vi "Mach1-TestRT-08-16.vi"() -> ()   [LabVIEW 2010]
uses:
  <vilib>/userDefined/High Color/nirio_resource_hc.ctl
  <vilib>/rvi/interface/nirviOpenFPGA/nirviOpenFPGA.xnode
  C:/Users/HAGAR-IV/Desktop/Zeugs/markus/version feb 2012/FPGA Bitfiles/pertrasgcfpga2_FPGATarget_Mach1-Test-08-16_84F9B2AA.lvbitx
  C:/Users/HAGAR-IV/Desktop/HAGAR-V_Steuerung/Users/HAGAR-IV/Desktop/Johnny/pertrasgc fpga/Mach1-Test-08-16.vi
  <vilib>/rvi/ClientSDK/nirviWhatTheDeviceIsDoing.ctl
  <vilib>/rvi/interface/nirviReadWriteControl/nirviReadWriteControl.xnode
  <vilib>/rvi/interface/common/niFpgaNodeNameForErrorReporting.ctl
  <vilib>/rvi/errors/niLvFpgaWhatHappensToTopLevelVI.ctl
  <vilib>/rvi/interface/nirviMethod/nirviMethod.xnode
  <vilib>/rvi/interface/nirviCloseFPGA/nirviCloseFPGA.xnode
  <vilib>/FPGAPlugInAG/cRIO-9114/niLvFpga_Open_cRIO-9114.vi
  <vilib>/rvi/interface/common/dynamic/niFpgaDynamicAddResources.vi
  <vilib>/Utility/error.llb/Error Cluster From Error Code.vi
  <vilib>/rvi/errors/niLvFpgaAdjustHostInterfaceError.vi
  <vilib>/FPGAPlugInAG/Dynamic/niLvFpga_Close_Dynamic.vi
  NiFpgaLv.dll
panel:
  in  "GrapfikLöschen":bool
  out "TempMach2":dbl[](graph)
  out "TempMach1":dbl[](graph)
  in  "2Pos1A":bool
  in  "Fan2":bool
  in  "Fan1":bool
  out "TempMach2":dbl
  out "TempMach1":dbl
  in  "KennlinieMach2":dbl[](array[numeric])=[-254.36, 617.83, -163.64]
  in  "TempMaxMach1":dbl format="%.14g"
  in  "TempMaxMach2":dbl format="%.14g"
  in  "PIDMach2":T1 {"proportional gain (Kc)" format="%.11g"; "integral gain (Kc*Ts/Ti)" format="%.11g"; "derivative gain (Kc*Td/Ts)" format="%.11g"}
  in  "PIDMach1":T1 {"proportional gain (Kc)" format="%.11g"; "integral gain (Kc*Ts/Ti)" format="%.11g"; "derivative gain (Kc*Td/Ts)" format="%.11g"}
  in  "Heizen?Mach2":bool
  in  "Heizen?Mach1":bool
  in  "Abstand zwischen Messungen [us]Mach":u16=20
  in  "wie viele Messwerte?Mach":u16=10
  in  "vor der Messung [us]Mach":u16=3000
  in  "Per[us]Mach":u16=30000
  in  "stop":bool
  in  "KennlinieMach1":dbl[](array[numeric])=[-247.14, 362.24, -56.76]
  in  "TempSPMach1":dbl format="%.14g"
  in  "TempSPMach2":dbl format="%.14g"
  # "Obacht: Hier gehts um\nPRE-MACH 1 und 2!!!"
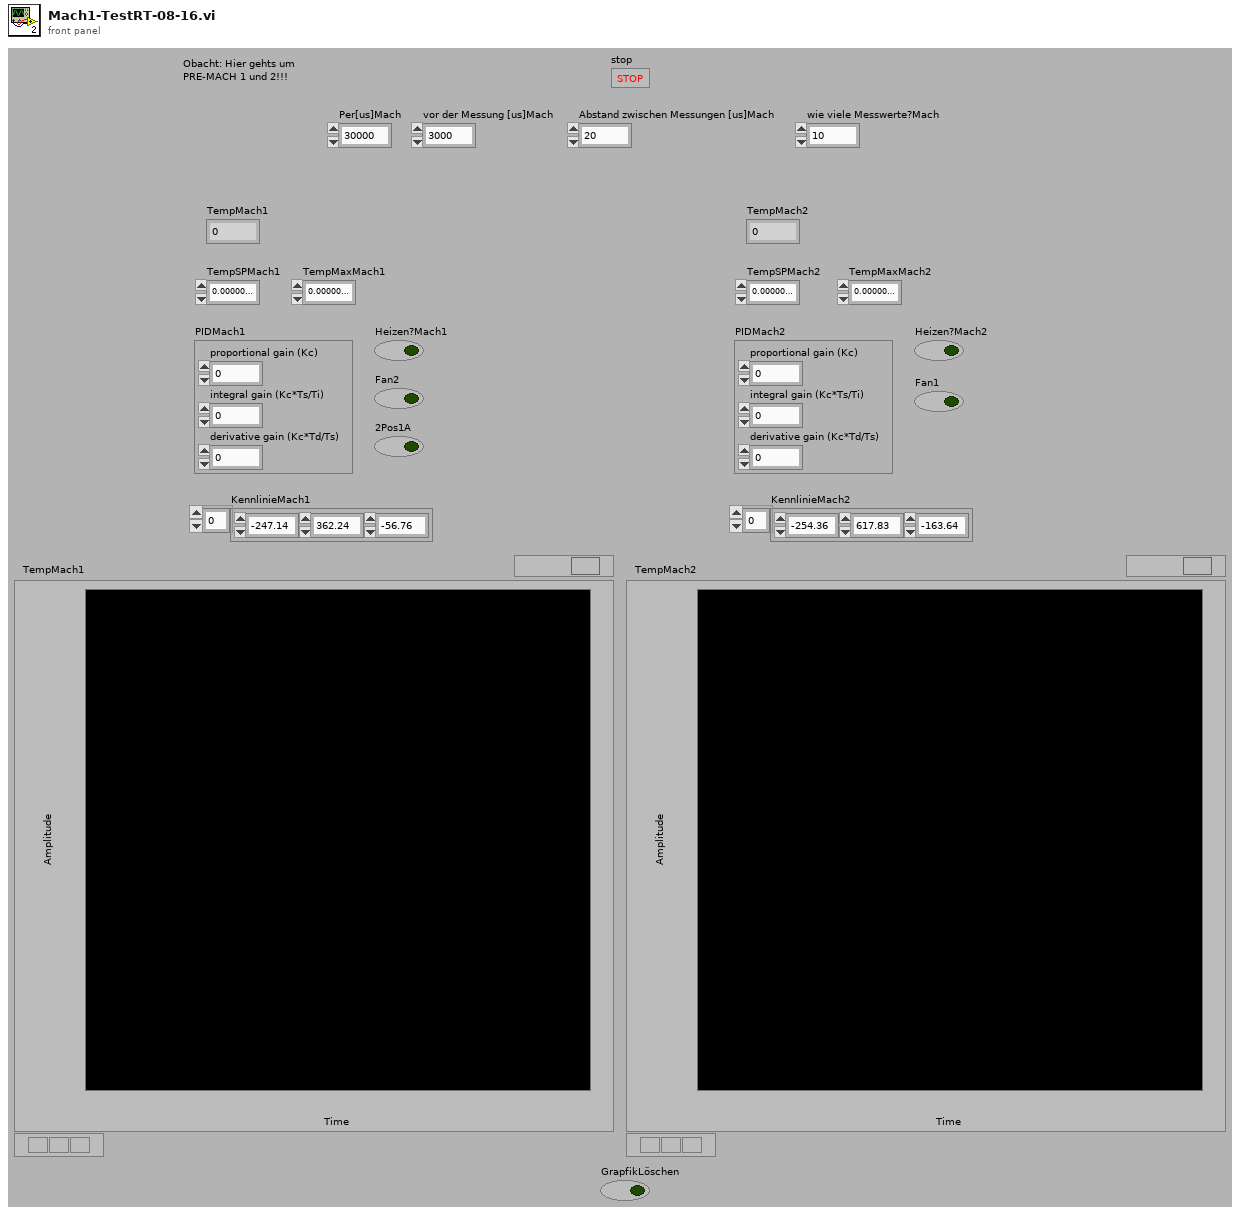
[diagram p1: front panel]
types:
  T1 = cluster{"proportional gain (Kc)":fxp<+/-,16,8>, "integral gain (Kc*Ts/Ti)":fxp<+/-,16,8>, "derivative gain (Kc*Td/Ts)":fxp<+/-,16,8>}
  T2 = typedef "niFpgaNodeNameForErrorReporting.ctl" = enum16{"Open FPGA VI Reference", "Read/Write Control", "Invoke Method: Abort", "Invoke Method: Acknowledge IRQ", "Invoke Method: Download", "Invoke Method: FIFO.Configure", "Invoke Method: FIFO.Read", "Invoke Method: FIFO.Start", "Invoke Method: FIFO.Stop", "Invoke Method: FIFO.Write", "Invoke Method: Reset", "Invoke Method: Run", "Invoke Method: Wait on IRQ", "Close FPGA VI Reference"}
  T3 = typedef "niLvFpgaWhatHappensToTopLevelVI.ctl" = enum16{"top level VI scripted behind XNode", "top level VI inlined behind XNode"}
  T4 = typedef "nirviWhatTheDeviceIsDoing.ctl" = enum32{"nothing", "something other than LabVIEW FPGA", "FPGA interface", "interactive", "emulation"}
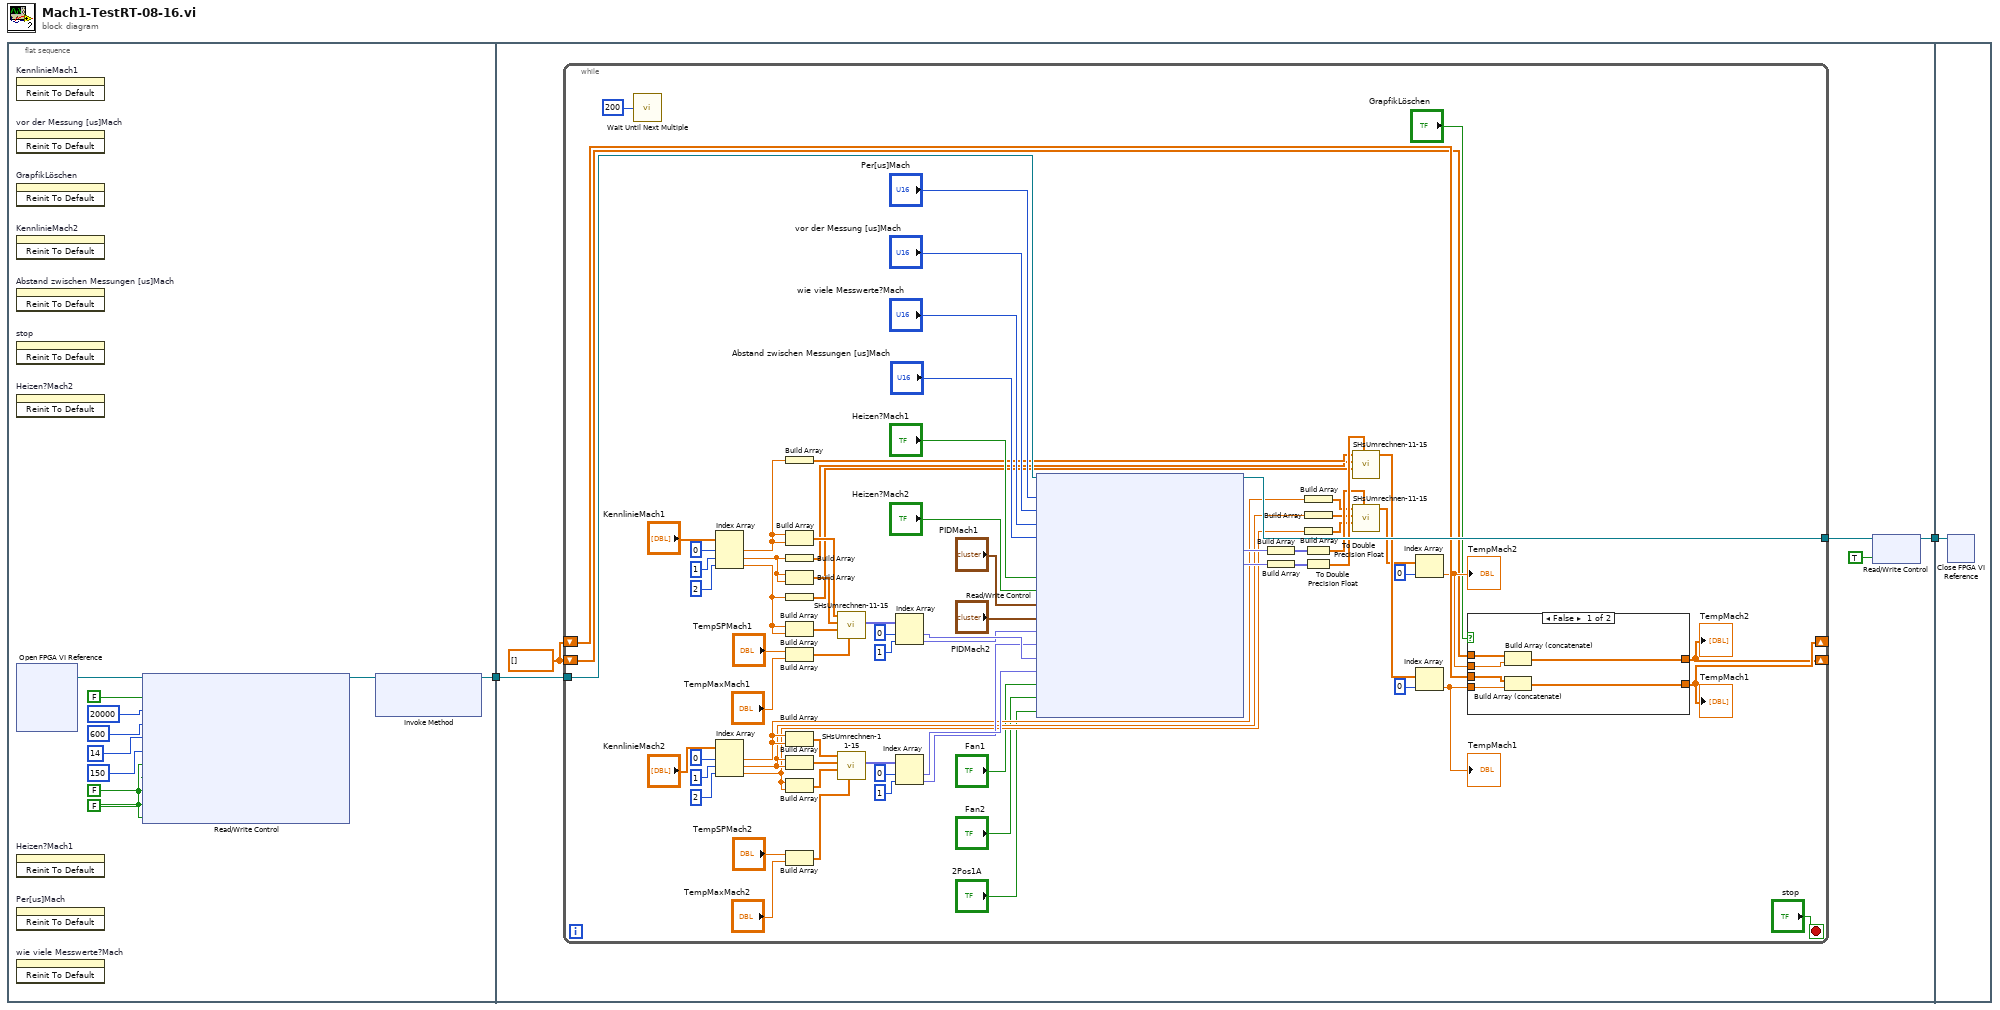
[diagram p0: block diagram]
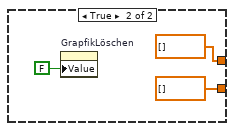
[diagram p2: hidden frame]
diagram:
  n1 = flat-sequence {
    tunnel: [w10] -> w2
    tunnel: w2 -> [w345]
    tunnel: [w342] -> w1
    tunnel: w1 -> [w913]
    frame #0 {
      w3 = FALSE ("Heizen?Mach2")
      n2 = invoke on="KennlinieMach1" class="Arr (strict)" method="Reinit To Default"() -> ()  [unwired: 3 in, 3 out]
      n3 = invoke on="vor der Messung [us]Mach" class="DigNum (strict)" method="Reinit To Default"() -> ()  [unwired: 3 in, 3 out]
      n4 = invoke on="GrapfikLöschen" class="Bool (strict)" method="Reinit To Default"() -> ()  [unwired: 3 in, 3 out]
      n5 = invoke on="KennlinieMach2" class="Arr (strict)" method="Reinit To Default"() -> ()  [unwired: 3 in, 3 out]
      n6 = invoke on="Abstand zwischen Messungen [us]Mach" class="DigNum (strict)" method="Reinit To Default"() -> ()  [unwired: 3 in, 3 out]
      n7 = invoke on="stop" class="Bool (strict)" method="Reinit To Default"() -> ()  [unwired: 3 in, 3 out]
      n8 = invoke on="Heizen?Mach2" class="Bool (strict)" method="Reinit To Default"() -> ()  [unwired: 3 in, 3 out]
      n9 = xnode "Open FPGA VI Reference"() -> ("FPGA VI Reference Out"=w12:refnum<k20>)  [unwired: 2 in, 1 out]
      n10 = invoke on="Heizen?Mach1" class="Bool (strict)" method="Reinit To Default"() -> ()  [unwired: 3 in, 3 out]
      n11 = invoke on="Per[us]Mach" class="DigNum (strict)" method="Reinit To Default"() -> ()  [unwired: 3 in, 3 out]
      n12 = invoke on="wie viele Messwerte?Mach" class="DigNum (strict)" method="Reinit To Default"() -> ()  [unwired: 3 in, 3 out]
      n13 = xnode "Read/Write Control"("FPGA VI Reference In"=w12, "stop"=FALSE, "Per[us]Mach"=u16 20000, "vor der Messung [us]Mach"=u16 600, "wie viele Messwerte?Mach"=u16 14, "Abstand zwischen Messungen [us]Mach"=u16 150, "Heizen?Mach1"=FALSE, "Heizen?Mach2"=w3, "Fan1"=w3, "Fan2"=w3, "2Pos1A"=w3) -> ("FPGA VI Reference Out"=w11:refnum<k20>)  [unwired: 1 in, 1 out]
      n14 = xnode "Invoke Method"("FPGA VI Reference In"=w11) -> ("FPGA VI Reference Out"=w10:refnum<k20>)  [unwired: 2 in, 1 out]
    }
    frame #1 {
      w341 = dbl[] []
      n15 = while {
        tunnel: w345 -> [w458]
        tunnel: [w457] -> w344
        shift-right: [w386] -> _
        shift-left: w341 -> [w390]
        shift-right: [w385] -> _
        shift-left: w341 -> [w388]
        stop <- "stop" stop-if-true
        n16 = call "Wait Until Next Multiple"("Count(mSec)"=u32 200) -> ()  [unwired: 1 out]
        n17 = Index Array(array="KennlinieMach1", index #1=0 ("index"), index #2=1 ("index"), index #3=2 ("index")) -> (element #1=w410:dbl, element #2=w409:dbl, element #3=w408:dbl)
        n18 = Index Array(array="KennlinieMach2", index #1=0 ("index"), index #2=1 ("index"), index #3=2 ("index")) -> (element #1=w402:dbl, element #2=w401:dbl, element #3=w400:dbl)
        n19 = Build Array(w410) -> (w407:dbl[])
        n20 = Build Array(w410, w410) -> (w426:dbl[])
        n21 = Build Array(w409) -> (w406:dbl[])
        n22 = Build Array(w409, w409) -> (w425:dbl[])
        n23 = Build Array(w408) -> (w405:dbl[])
        n24 = Build Array(w408, w408) -> (w424:dbl[])
        n25 = Build Array("TempSPMach1", "TempMaxMach1") -> (w444:dbl[])
        n26 = Build Array(w402, w402) -> (w419:dbl[])
        n27 = Build Array(w401, w401) -> (w418:dbl[])
        n28 = Build Array(w400, w400) -> (w417:dbl[])
        n29 = Build Array("TempSPMach2", "TempMaxMach2") -> (w436:dbl[])
        n30 = call "SHsUmrechnen-11-15.vi"("TemperaturenSH[V]"=w444, "Traps/MachKoeff2"=w424, "Traps/MachKoeff1"=w425, "Traps/MachKoeff0"=w426) -> ("SpannungenSH[V]"=w443:fxp<+/-,16,4>[])  [unwired: 6 in, 1 out]
        n31 = call "SHsUmrechnen-11-15.vi"("TemperaturenSH[V]"=w436, "Traps/MachKoeff2"=w417, "Traps/MachKoeff1"=w418, "Traps/MachKoeff0"=w419) -> ("SpannungenSH[V]"=w433:fxp<+/-,16,4>[])  [unwired: 6 in, 1 out]
        n32 = Index Array(array=w443, index #1=0 ("index"), index #2=1 ("index")) -> (element #1=w440:fxp<+/-,16,4>, element #2=w439:fxp<+/-,16,4>)
        n33 = Index Array(array=w433, index #1=0 ("index"), index #2=1 ("index")) -> (element #1=w432:fxp<+/-,16,4>, element #2=w431:fxp<+/-,16,4>)
        n34 = xnode "Read/Write Control"("FPGA VI Reference In"=w458, "Per[us]Mach"="Per[us]Mach", "vor der Messung [us]Mach"="vor der Messung [us]Mach", "wie viele Messwerte?Mach"="wie viele Messwerte?Mach", "Abstand zwischen Messungen [us]Mach"="Abstand zwischen Messungen [us]Mach", "Heizen?Mach1"="Heizen?Mach1", "Heizen?Mach2"="Heizen?Mach2", "PIDMach1"="PIDMach1", "PIDMach2"="PIDMach2", "Umax[V]Mach1"=w439, "Umax[V]Mach2"=w431, "USetp[V]Mach1"=w440, "USetp[V]Mach2"=w432, "Fan1"="Fan1", "Fan2"="Fan2", "2Pos1A"="2Pos1A") -> ("FPGA VI Reference Out"=w457:refnum<k20>, "U[V]Mach2"=w412:fxp<+/-,16,4>, "U[V]Mach1"=w416:fxp<+/-,16,4>)  [unwired: 1 in, 1 out]
        n35 = Build Array(w412) -> (w413:fxp<+/-,16,4>[])
        n36 = Build Array(w416) -> (w415:fxp<+/-,16,4>[])
        n37 = Build Array(w402) -> (w399:dbl[])
        n38 = Build Array(w401) -> (w398:dbl[])
        n39 = Build Array(w400) -> (w397:dbl[])
        n40 = To Double Precision Float(number=w413) -> (double precision float=w411:dbl[])
        n41 = To Double Precision Float(number=w415) -> (double precision float=w414:dbl[])
        n42 = call "SHsUmrechnen-11-15.vi"("SpannungenSH[V]"=w414, "Traps/MachKoeff2"=w405, "Traps/MachKoeff1"=w406, "Traps/MachKoeff0"=w407) -> ("TemperaturenSH[°C]"=w404:dbl[])  [unwired: 6 in, 1 out]
        n43 = call "SHsUmrechnen-11-15.vi"("SpannungenSH[V]"=w411, "Traps/MachKoeff2"=w397, "Traps/MachKoeff1"=w398, "Traps/MachKoeff0"=w399) -> ("TemperaturenSH[°C]"=w395:dbl[])  [unwired: 6 in, 1 out]
        n44 = Index Array(array=w395, index=0) -> (element=w389:dbl)
        "TempMach2" <- w389
        n45 = Index Array(array=w404, index=0) -> (element=w391:dbl)
        "TempMach1" <- w391
        n46 = case shown="False" "GrapfikLöschen" {
          tunnel: w391 -> [w464 _]
          tunnel: [w463 dbl[] []] -> w386
          tunnel: w390 -> [w462 _]
          tunnel: w389 -> [w461 _]
          tunnel: [w460 dbl[] []] -> w385
          tunnel: w388 -> [w459 _]
          frame False {
            n47 = Build Array (concatenate)(w459, w461) -> (w460:dbl[])
            n48 = Build Array (concatenate)(w462, w464) -> (w463:dbl[])
          }
          frame True {
            n49 = property on="GrapfikLöschen" class="Bool (strict)"("Value"=FALSE ("GrapfikLöschen")) -> ()  [unwired: 2 in, 2 out]
          }
        }
        "TempMach1" <- w386
        "TempMach2" <- w385
      }
      n50 = xnode "Read/Write Control"("FPGA VI Reference In"=w344, "stop"=TRUE) -> ("FPGA VI Reference Out"=w342:refnum<k20>)  [unwired: 1 in, 1 out]
    }
    frame #2 {
      n51 = xnode "Close FPGA VI Reference"("FPGA VI Reference In"=w913) -> ()  [unwired: 1 in, 1 out]
    }
  }
